vi "Overwrite-all-hidden-params.vi"(8 "error in (no error)":errorcluster, 10 "Correct params adv":T1={"2nd image mirror axis"=1, "Cross-correlation decimation"=5, "Cross-correlation algorithm"=enum."frequency domain", "Always threshold when smoothing?"=TRUE, "Threshold only 2nd camera image?"=TRUE, "Median filter type"={"Order #"=4, "Y Size"=3, "X Size"=3}, "Gaussian filter kernel size"=3, "Gaussian filter kernel number"=3}, 11 "Correct. params. ref. in":refnum<data-value>) -> (0 "error out":errorcluster, 3 "Correct. params. ref.":refnum<data-value>)   [LabVIEW 2013, in "CameraVision.lvlib" / "CV-Correction.lvclass"]
uses:
  CV-Correction.lvclass
  Correction-parameters-advanced.ctl
  CV-Correction.lvclass/CV-Correction.ctl
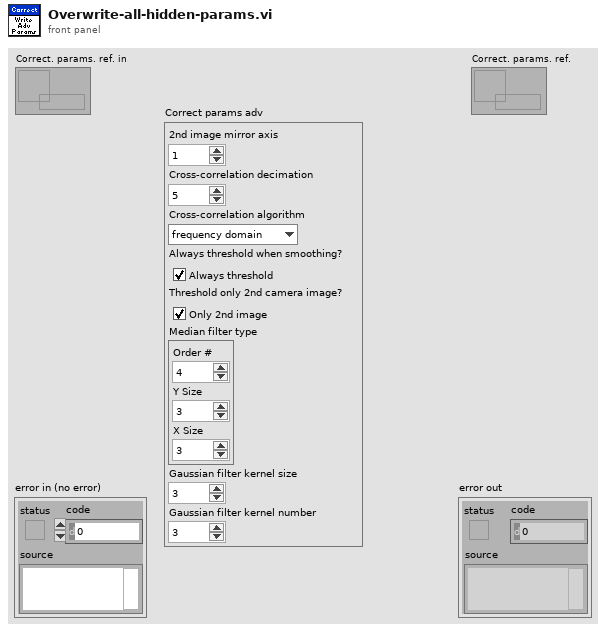
[diagram p1: front panel]
types:
  T1 = typedef "CameraVision.lvlib/CV-Correction.lvclass/Correction-parameters-advanced.ctl" = cluster{"2nd image mirror axis":u32, "Cross-correlation decimation":i32, "Cross-correlation algorithm":enum32{"direct", "frequency domain"}, "Always threshold when smoothing?":bool, "Threshold only 2nd camera image?":bool, "Median filter type":cluster{"Order #":i32, "Y Size":i32, "X Size":i32}, "Gaussian filter kernel size":i32, "Gaussian filter kernel number":i32}
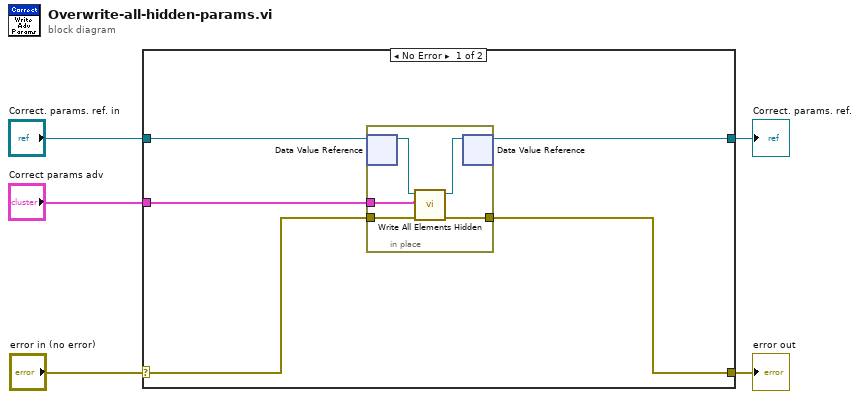
[diagram p0: block diagram]
diagram:
  n1 = case shown="No Error" "error in (no error)" {
    selector: "error in (no error)" -> [w8 w17]
    tunnel: [w9 w17] -> w4
    tunnel: "Correct. params. ref. in" -> [w7 w16]
    tunnel: "Correct params adv" -> [w10 _]
    tunnel: [w6 w16] -> w1
    frame No Error {
      n2 = in-place {
        in-place-border: w10 -> [w15]
        in-place-border: [w14] -> w9
        in-place-border: w8 -> [w13]
        n3 = in-place-dvr #1(w7) -> (w11:refnum<class "CV-Correction.lvclass">)  [unwired: 1 out]
        n4 = call "Write All Elements Hidden.vi"("error in (no error)"=w13, "Correct. params. hidden"=w15, "Correct params in"=w11) -> ("error out"=w14:errorcluster, "Correct params out"=w12:refnum<class "CV-Correction.lvclass">)  [unwired: 7 in]
        n5 = in-place-dvr #1(w12) -> (w6:refnum<data-value>)  [unwired: 1 out]
      }
    }
    frame Error {
    }
  }
  "error out" <- w4
  "Correct. params. ref." <- w1
